vi "Get Target t0.vi"(11 "Analog Waveform Array in":waveform(dbl)[](array[waveform])) -> (3 "Target t0":timestamp)   [LabVIEW 2018, in "Waveform Equalizer.lvlib"]
uses:
  Waveform Equalizer.lvlib
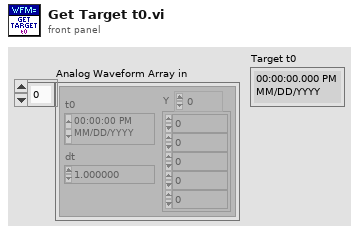
[diagram p1: front panel]
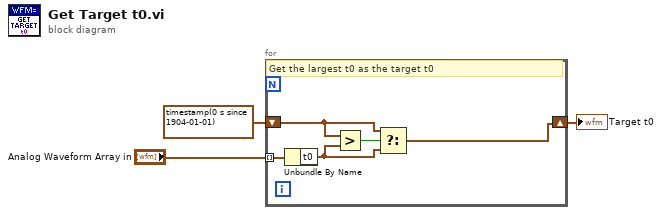
[diagram p0: block diagram]
diagram:
  n1 = for {
    tunnel: "Analog Waveform Array in" -> [w8] mode=indexing
    shift-right: [w4] -> w3
    shift-left: timestamp(0 s since 1904-01-01) -> [w6]
    # "Get the largest t0 as the target t0"
    n2 = Unbundle By Name(w8) -> ("t0"=w5:timestamp)
    n3 = Greater?(x=w6, y=w5) -> (0:w7:bool)
    n4 = Select(t=w6, s=w7, f=w5) -> (s? t:f=w4:timestamp)
  }
  "Target t0" <- w3
